vi "TEST_TRAJECTORY_EXECUTE_SWERVE.vi"(6 "EnableClosedLoop":bool=TRUE, 7 "Orientation Dmd In":dbl, 8 "Init":bool=TRUE, 9 "Reverse":bool, 10 "Follow Orientation":bool) -> (0 "AtReference":bool, 3 "Chassis Velocity Target":T2 {"vOmega" format="%10.3f"; "vY" format="%10.3f"; "vX" format="%10.3f"}, 4 "Time Offset":dbl=-1.0 format="%16.4f", 5 "Orientation Target":dbl, 11 "Gyro Heading":dbl)   [LabVIEW 2019]
uses:
  <vilib>/Rock Robotics/WPI/ThirdParty/JAS_Junk/TrajLib/Trajectory_Library.lvlib
  <vilib>/Rock Robotics/WPI/ThirdParty/JAS_Junk/TrajLib/TypeDef/CHASSIS_SPEEDS.ctl
  Swerve_Drive_System/SDO_DRIVE_GLOBALS.vi
  Simulation/SDO_SIM_SIM_Globals.vi
  <vilib>/Rock Robotics/WPI/ThirdParty/JAS_Junk/TrajLib/TypeDef/TRANSLATION2D.ctl
  <vilib>/Rock Robotics/WPI/ThirdParty/JAS_Junk/TrajLib/TypeDef/ROTATION2D.ctl
  <vilib>/Rock Robotics/WPI/ThirdParty/JAS_Junk/TrajLib/TypeDef/POSE2D.ctl
  <vilib>/Rock Robotics/WPI/ThirdParty/JAS_Junk/TrajLib/TypeDef/TRAJ_STATE.ctl
panel:
  in  "Tab Control":T1(tab)
  out "OutputTRAJ_STATE":T3={"TimeSeconds"=0.0, "Velocity"=0.0, "Acceleration"=0.0, "POSE"={"TRANSLATION"={"X"=0.0, "Y"=0.0}, "ROTATION"={"VALUE"=0.0, "COS"=1.0, "SIN"=0.0}}, "Curvature"=0.0} {"POSE"."ROTATION"."SIN" format="%13.4f"; "POSE"."ROTATION"."COS" format="%13.4f"; "POSE"."ROTATION"."VALUE" format="%13.4f"; "POSE"."TRANSLATION"."Y" format="%14.3f"; "POSE"."TRANSLATION"."X" format="%14.3f"}
  in  "Step":bool
  in  "Trajectory File Name":path=path "Sample-Robot-2-Trajectory-TrajLibrary.csv"
  out "Traj File Good":bool
  out "Module Ang\nRadians":dbl
  out "Module Speed\nM/S":dbl
  in  "Run":bool
  out "Rel Odom":T4={"TRANSLATION"={"X"=0.0, "Y"=0.0}, "ROTATION"={"VALUE"=0.0, "COS"=1.0, "SIN"=0.0}} {"ROTATION"."SIN" format="%13.4f"; "ROTATION"."COS" format="%13.4f"; "ROTATION"."VALUE" format="%13.4f"; "TRANSLATION"."Y" format="%14.3f"; "TRANSLATION"."X" format="%14.3f"}
  out "Error and Corr":T7 {"Error Pose"."ROTATION"."SIN" format="%13.4f"; "Error Pose"."ROTATION"."COS" format="%13.4f"; "Error Pose"."ROTATION"."VALUE" format="%13.4f"; "Error Pose"."TRANSLATION"."Y" format="%14.3f"; "Error Pose"."TRANSLATION"."X" format="%14.3f"}
  out "Abs Odom":T4={"TRANSLATION"={"X"=0.0, "Y"=0.0}, "ROTATION"={"VALUE"=0.0, "COS"=1.0, "SIN"=0.0}} {"ROTATION"."SIN" format="%13.4f"; "ROTATION"."COS" format="%13.4f"; "ROTATION"."VALUE" format="%13.4f"; "TRANSLATION"."Y" format="%14.3f"; "TRANSLATION"."X" format="%14.3f"}
  out "Traj Err":cluster{"X":dbl, "Y":dbl, "Angle":dbl}(graph)
  out "Traj Correction":cluster{"X Corr":dbl, "Y Corr":dbl}(graph)
  out "Robot Position":cluster{dbl[], dbl[]}(graph)
  # "Module States"
  # "For now all modules use this value..."
  # "(FOR TESTING)"
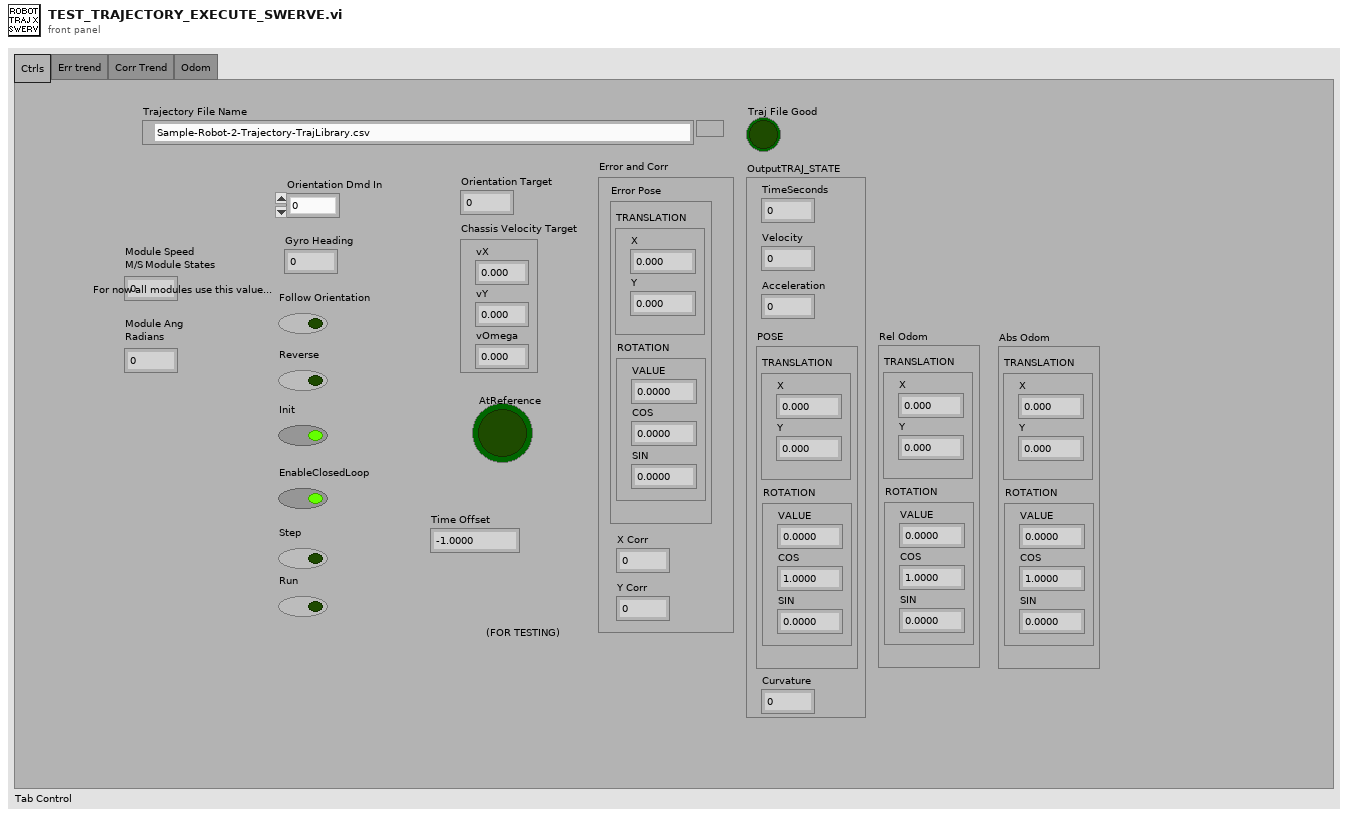
[diagram p1: front panel]
types:
  T1 = enum32{"Ctrls", "Err trend", "Corr Trend", "Odom"}
  T2 = typedef "Trajectory_Library.lvlib/CHASSIS_SPEEDS.ctl" = cluster{"vX":dbl, "vY":dbl, "vOmega":dbl}
  T3 = typedef "Trajectory_Library.lvlib/TRAJ_STATE.ctl" = cluster{"TimeSeconds":dbl, "Velocity":dbl, "Acceleration":dbl, "POSE":T4, "Curvature":dbl}
  T4 = typedef "Trajectory_Library.lvlib/POSE2D.ctl" = cluster{"TRANSLATION":T5, "ROTATION":T6}
  T5 = typedef "Trajectory_Library.lvlib/TRANSLATION2D.ctl" = cluster{"X":dbl, "Y":dbl}
  T6 = typedef "Trajectory_Library.lvlib/ROTATION2D.ctl" = cluster{"VALUE":dbl, "COS":dbl, "SIN":dbl}
  T7 = cluster{"Error Pose":T4, "X Corr":dbl, "Y Corr":dbl}
  T8 = typedef "Trajectory_Library.lvlib/SWERVE_DRIVE_MODULE_POSITION.ctl" = cluster{"Distance":dbl, "Angle":T6, "P":bool}
  T9 = typedef "Trajectory_Library.lvlib/SWERVE_DRIVE_ODOMETRY.ctl" = cluster{"POSE":T4, "GyroOffset":T6, "PreviousAngle":T6, "PrevModulePositions":T8[], "NumModules":i32}
  T10 = typedef "Trajectory_Library.lvlib/SWERVE_DRIVE_KINEMATICS.ctl" = cluster{"NumModules":i32, "InverseKinematics":T11, "ForwardKinematics":T11, "Modules":T5[], "PrevCoR":T5, "SavedModuleStates":T12[]}
  T11 = typedef "NI_Matrix.lvlib/RealMatrix.ctl" = dbl[][]
  T12 = typedef "Trajectory_Library.lvlib/SWERVE_DRIVE_MODULE_STATE.ctl" = cluster{"Speed":dbl, "Angle":T6}
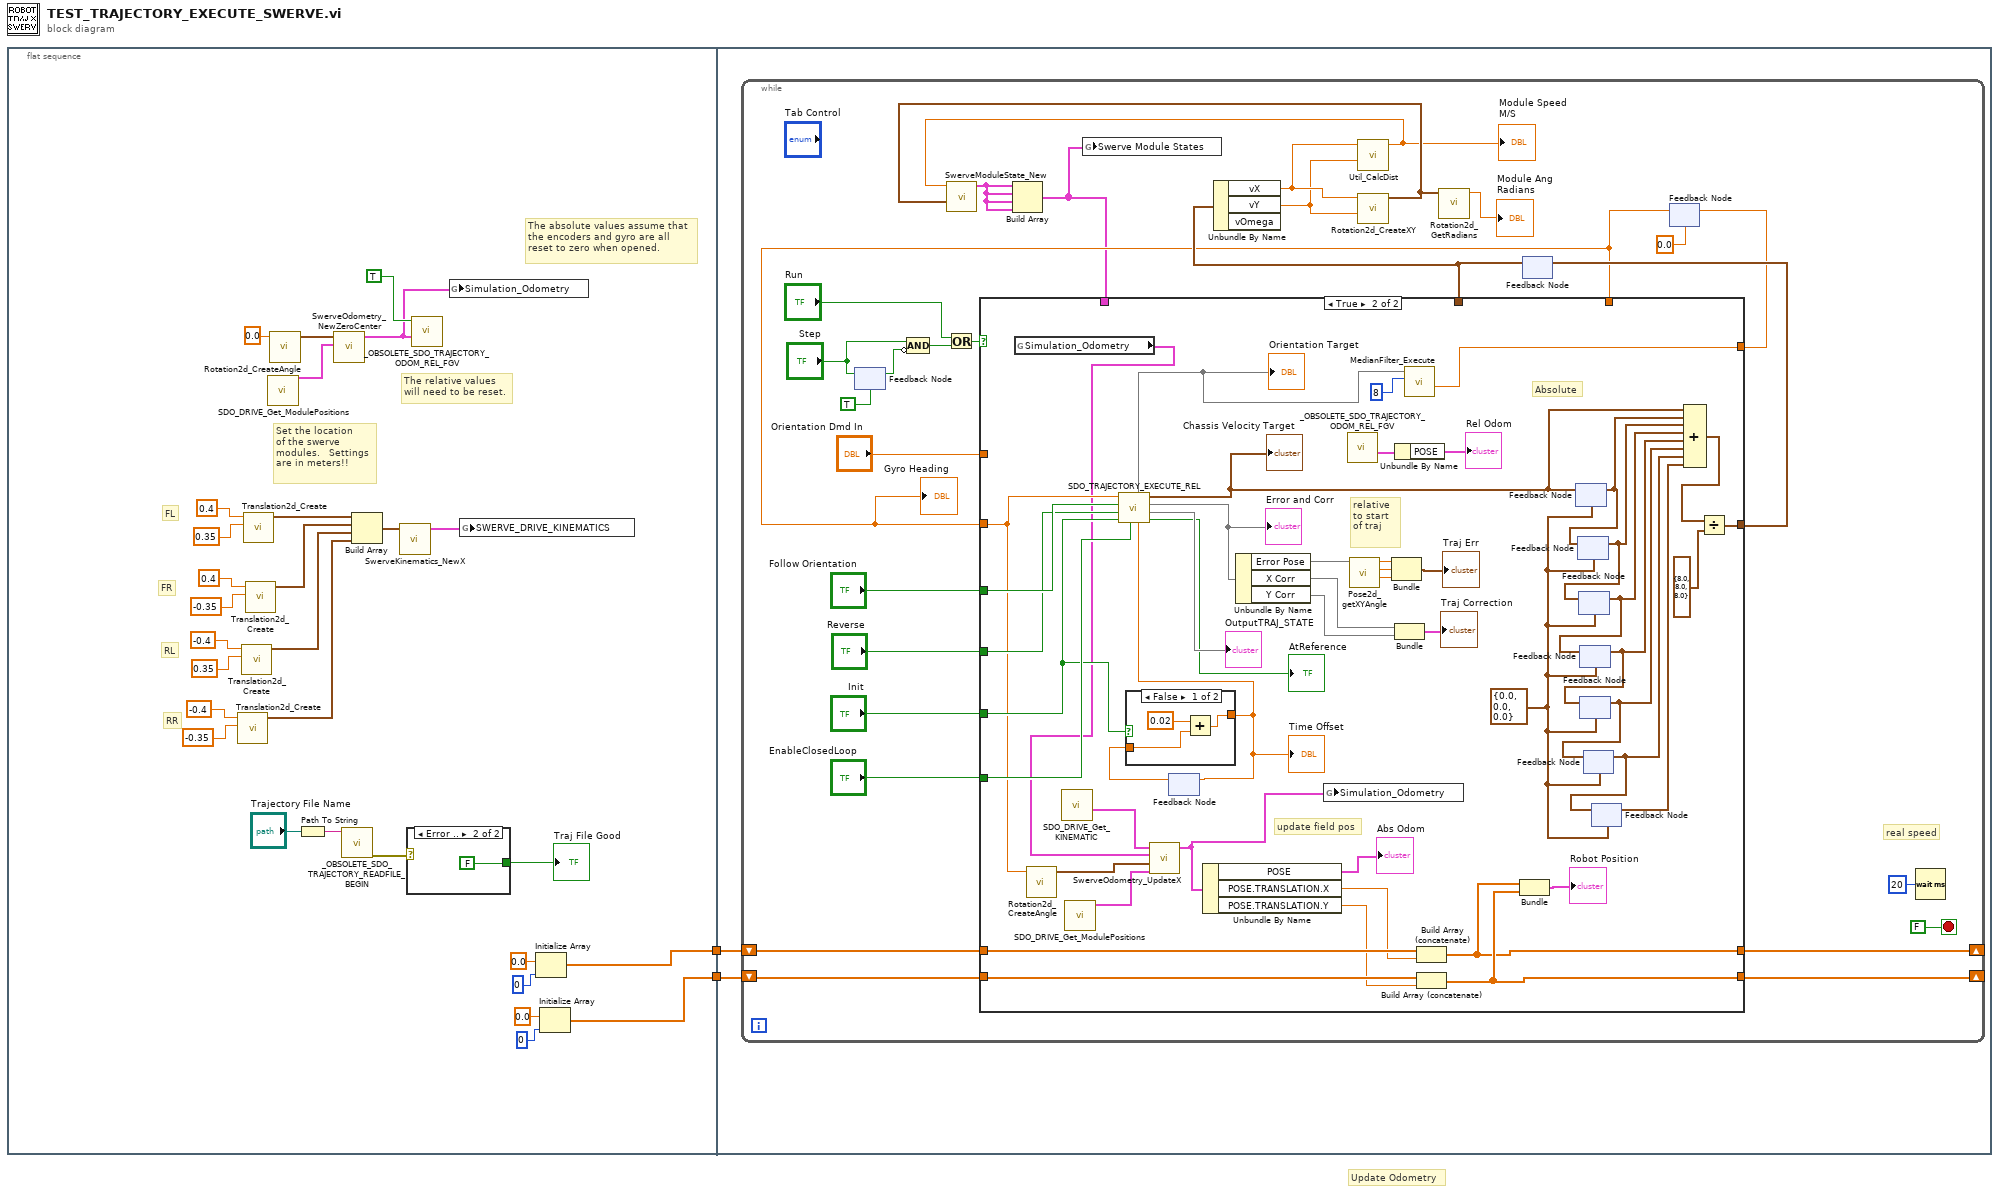
[diagram p0: block diagram]
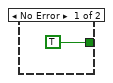
[diagram p2: hidden frame]
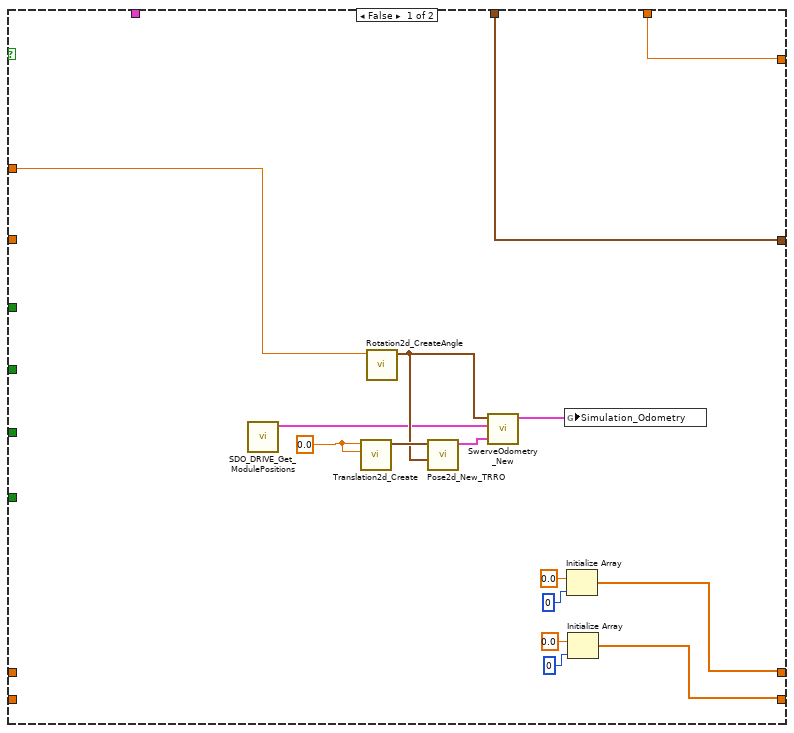
[diagram p3: hidden frame]
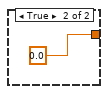
[diagram p4: hidden frame]
diagram:
  # "Update Odometry"
  n1 = flat-sequence {
    tunnel: [w10] -> w2
    tunnel: [w7] -> w1
    tunnel: w2 -> [w35]
    tunnel: w1 -> [w34]
    frame #0 {
      # "The absolute values assume that\nthe encoders and gyro are all\nreset to zero when opened."
      # "RR"
      # "RL"
      # "FR"
      # "FL"
      # "Set the location\nof the swerve \nmodules.   Settings\nare in meters!!"
      # "The relative values\nwill need to be reset."
      n2 = call <vilib>:"Translation2d_Create.vi"("Y"=-0.35, "X"=-0.4) -> ("TRANSLATION"=w13:T5)  [unwired: 9 in]
      n3 = call <vilib>:"Translation2d_Create.vi"("Y"=0.35, "X"=-0.4) -> ("TRANSLATION"=w17:T5)  [unwired: 9 in]
      n4 = call <vilib>:"Translation2d_Create.vi"("Y"=0.35, "X"=0.4) -> ("TRANSLATION"=w19:T5)  [unwired: 9 in]
      n5 = call <vilib>:"Translation2d_Create.vi"("Y"=-0.35, "X"=0.4) -> ("TRANSLATION"=w18:T5)  [unwired: 9 in]
      n6 = call "SDO_DRIVE_Get_ModulePositions.vi"() -> ("Swerve Module Positions"=w5:T8[])  [unwired: 11 in]
      n7 = call <vilib>:"Rotation2d_CreateAngle.vi"("Angle"=0.0) -> ("ROTATION"=w26:T6)  [unwired: 10 in]
      n8 = Path To String(path="Trajectory File Name") -> (string=w30:string)
      n9 = call <vilib>:"SwerveOdometry_NewZeroCenter.vi"("Module Positions"=w5, "gyroAngle"=w26) -> ("SWERVE_DRIVE_ODOMETRY"=w3:T9)  [unwired: 9 in]
      n10 = call "_OBSOLETE_SDO_TRAJECTORY_READFILE_BEGIN.vi"("Trajectory File Name"=w30) -> ("error out"=w31:errorcluster)  [unwired: 7 in, 3 out]
      n11 = Build Array(w19, w18, w17, w13) -> (w16:T5[])
      n12 = call <vilib>:"SwerveKinematics_NewX.vi"("Wheels"=w16) -> ("SWERVE_DRIVE_KINEMATICS"=w4:T10)  [unwired: 10 in]
      n13 = case shown="Error .." w31 {
        tunnel: [TRUE FALSE] -> w28
        frame No Error {
        }
        frame Error {
        }
      }
      "Traj File Good" <- w28
      n14 = call "_OBSOLETE_SDO_TRAJECTORY_ODOM_REL_FGV.vi"("in SWERVE_DRIVE_ODOMETRY"=w3, "WRITE"=TRUE) -> ()  [unwired: 9 in, 1 out]
      n15 = global write "SDO_SIM_SIM_Globals.vi" "Simulation_Odometry"(w3) -> ()
      n16 = global write "SDO_DRIVE_GLOBALS.vi" "SWERVE_DRIVE_KINEMATICS"(w4) -> ()
      n17 = Initialize Array(0.0 ("element"), 0 ("dimension size")) -> (w10:dbl[])
      n18 = Initialize Array(0.0 ("element"), 0 ("dimension size")) -> (w7:dbl[])
    }
    frame #1 {
      n19 = while {
        shift-right: [w37] -> _
        shift-left: w35 -> [w40]
        shift-right: [w38] -> _
        shift-left: w34 -> [w39]
        stop <- FALSE stop-if-true
        # "real speed"
        n20 = feedback #1(TRUE ("Step")) -> (w61:bool)
        n21 = feedback-in #1("Step") -> ()
        n22 = Compound Arithmetic op=AND("Step", invert w61) -> (w47:bool)
        n23 = Or(x="Run", y=w47) -> (x .or. y?=w46:bool)
        n24 = feedback #2() -> (w53:T2)  [unwired: 1 in]
        n25 = Unbundle By Name(w53) -> ("vX"=w52:dbl, "vY"=w51:dbl)  [unwired: 1 out]
        n26 = call <vilib>:"Util_CalcDist.vi"("Y"=w51, "X"=w52) -> ("DIST"=w48:dbl)  [unwired: 9 in]
        "Module Speed\nM/S" <- w48
        n27 = call <vilib>:"Rotation2d_CreateXY.vi"("Y or sine"=w51, "X or  cosine"=w52) -> ("ROTATION"=w50:T6)  [unwired: 9 in]
        n28 = call <vilib>:"SwerveModuleState_New.vi"("ROTATION"=w50, "Speed"=w48) -> ("SWERVE_DRIVE_MODULE_STATE"=w56:T12)  [unwired: 9 in]
        n29 = Build Array(w56, w56, w56, w56) -> (w36:T12[])
        n30 = global write "SDO_DRIVE_GLOBALS.vi" "Swerve Module States"(w36) -> ()
        n31 = call <vilib>:"Rotation2d_GetRadians.vi"("in ROTATION"=w50) -> ("AngleRadians"=→"Module Ang\nRadians":dbl)  [unwired: 10 in]
        n32 = feedback #3(0.0 ("MedianValue")) -> (w42:dbl)
        "Gyro Heading" <- w42
        n33 = case shown="True" w46 {
          tunnel: w42 -> [_ w86]
          tunnel: "Follow Orientation" -> [_ w127]
          tunnel: "Reverse" -> [_ w126]
          tunnel: "Init" -> [_ w121]
          tunnel: "EnableClosedLoop" -> [_ w125]
          tunnel: "Orientation Dmd In" -> [w71 _]
          tunnel: w36 -> [_ _]
          tunnel: [w79 w108] -> w54
          tunnel: w53 -> [w79 _]
          tunnel: [w78 w101] -> w44
          tunnel: w42 -> [w78 _]
          tunnel: w40 -> [_ w92]
          tunnel: w39 -> [_ w93]
          tunnel: [w75 w90] -> w38
          tunnel: [w72 w89] -> w37
          frame False {
            w69 = 0.0 ("X")
            n34 = call "SDO_DRIVE_Get_ModulePositions.vi"() -> ("Swerve Module Positions"=w66:T8[])  [unwired: 11 in]
            n35 = call <vilib>:"Translation2d_Create.vi"("Y"=w69, "X"=w69) -> ("TRANSLATION"=w70:T5)  [unwired: 9 in]
            n36 = call <vilib>:"Rotation2d_CreateAngle.vi"("Angle"=w71) -> ("ROTATION"=w68:T6)  [unwired: 10 in]
            n37 = call <vilib>:"Pose2d_New_TRRO.vi"("ROTATION"=w68, "TRANSLATION"=w70) -> ("outPOSE"=w67:T4)  [unwired: 9 in]
            n38 = call <vilib>:"SwerveOdometry_New.vi"("InitialPose"=w67, "Module Positions"=w66, "gyroAngle"=w68) -> ("SWERVE_DRIVE_ODOMETRY"=w65:T9)  [unwired: 8 in]
            n39 = global write "SDO_SIM_SIM_Globals.vi" "Simulation_Odometry"(w65) -> ()
            n40 = Initialize Array(0.0 ("element"), 0 ("dimension size")) -> (w72:dbl[])
            n41 = Initialize Array(0.0 ("element"), 0 ("dimension size")) -> (w75:dbl[])
          }
          frame True {
            w119 = T2 {"vX"=0.0, "vY"=0.0, "vOmega"=0.0} ("Chassis Velocity Target")
            # "update field pos"
            # "Absolute"
            # "relative to start of traj"
            n42 = global read "SDO_SIM_SIM_Globals.vi" "Simulation_Odometry"() -> (w80:T9)
            n43 = call <vilib>:"Rotation2d_CreateAngle.vi"("Angle"=w86) -> ("ROTATION"=w83:T6)  [unwired: 10 in]
            n44 = call "SDO_DRIVE_Get_KINEMATIC.vi"() -> ("out SWERVE_DRIVE_KINEMATICS"=w84:T10)  [unwired: 11 in]
            n45 = call "SDO_DRIVE_Get_ModulePositions.vi"() -> ("Swerve Module Positions"=w82:T8[])  [unwired: 11 in]
            n46 = call <vilib>:"SwerveOdometry_UpdateX.vi"("module Positions"=w82, "gyroAngle"=w83, "in SWERVE_DRIVE_ODOMETRY"=w80, "SWERVE_DRIVE_KINEMATICS"=w84) -> ("out SWERVE_DRIVE_ODOMETRY"=w81:T9)  [unwired: 5 in, 2 out]
            n47 = feedback #4() -> (w122:dbl)  [unwired: 1 in]
            n48 = case shown="False" w121 {
              tunnel: [w130 0.0] -> w120
              tunnel: w122 -> [w128 _]
              frame False {
                n49 = Add(x=0.02, y=w128) -> (x+y=w130:dbl)
              }
              frame True {
              }
            }
            "Time Offset" <- w120
            n50 = call "SDO_TRAJECTORY_EXECUTE_REL.vi"(4:w120, "EnableClosedLoop"=w125, "Init"=w121, "Reverse"=w126, "End Relative\nOrientation Deg"=w127, "Gyro Heading\nRAD"=w86) -> ("AtReference"=→"AtReference":bool, 1:→"OutputTRAJ_STATE", 2:w100, "Chassis Velocity Target"=w118:T2, 5:w103)  [unwired: 1 in]
            "Orientation Target" <- w103
            "Chassis Velocity Target" <- w118
            "Error and Corr" <- w100
            n51 = feedback-in #4(w120) -> ()
            n52 = Unbundle By Name(w81) -> ("POSE"=→"Abs Odom":T4, "POSE.TRANSLATION.X"=w88:dbl, "POSE.TRANSLATION.Y"=w87:dbl)
            n53 = Unbundle By Name(w100) -> ("Error Pose"=w99, "X Corr"=w98, "Y Corr"=w97)
            n54 = global write "SDO_SIM_SIM_Globals.vi" "Simulation_Odometry"(w81) -> ()
            n55 = call "_OBSOLETE_SDO_TRAJECTORY_ODOM_REL_FGV.vi"() -> ("out SWERVE_DRIVE_ODOMETRY"=w94:T9)  [unwired: 11 in]
            n56 = call <vilib>:"Pose2d_getXYAngle.vi"("in POSE"=w99) -> ("Angle"=w104:dbl, "Y"=w105:dbl, "X"=w106:dbl)  [unwired: 8 in]
            n57 = Bundle("X"=w106, "Y"=w105, "Angle"=w104) -> (→"Traj Err":cluster{"X":dbl, "Y":dbl, "Angle":dbl})  [unwired: 1 in]
            n58 = Unbundle By Name(w94) -> ("POSE"=→"Rel Odom":T4)
            n59 = Bundle("X Corr"=w98, "Y Corr"=w97) -> (→"Traj Correction":cluster{"X Corr":void, "Y Corr":void})  [unwired: 1 in]
            n60 = call <vilib>:"MedianFilter_Execute.vi"("Samples"=8, "Input Value"=w103) -> ("MedianValue"=w101:dbl)  [unwired: 8 in, 1 out]
            n61 = Build Array (concatenate)(w92, w88) -> (w89:dbl[])
            n62 = Build Array (concatenate)(w93, w87) -> (w90:dbl[])
            n63 = Bundle(w89, w90) -> (→"Robot Position":cluster{dbl[], dbl[]})  [unwired: 1 in]
            n64 = feedback-in #5(w118) -> ()
            n65 = feedback #5(w119) -> (w117:T2)
            n66 = feedback #6(w119) -> (w116:T2)
            n67 = feedback-in #6(w117) -> ()
            n68 = feedback #7(w119) -> (w115:T2)
            n69 = feedback-in #7(w116) -> ()
            n70 = feedback #8(w119) -> (w114:T2)
            n71 = feedback-in #8(w115) -> ()
            n72 = feedback #9(w119) -> (w113:T2)
            n73 = feedback-in #9(w114) -> ()
            n74 = feedback #10(w119) -> (w112:T2)
            n75 = feedback-in #10(w113) -> ()
            n76 = feedback #11(w119) -> (w111:T2)
            n77 = feedback-in #11(w112) -> ()
            n78 = Compound Arithmetic op=ADD(w118, w117, w116, w115, w114, w113, w112, w111) -> (w110:T2)
            n79 = Divide(x=w110, y=T2 {"vX"=8.0, "vY"=8.0, "vOmega"=8.0}) -> (x/y=w108:T2)
          }
        }
        n80 = feedback-in #2(w54) -> ()
        n81 = feedback-in #3(w44) -> ()
        n82 = Wait (ms)(milliseconds to wait=u32 20) -> ()  [unwired: 1 out]
      }
    }
  }
